vi "GVSGet QueueName From DataView Idx.vi"(11 "DataView Idx":i32) -> (3 "DataView sQueueName":string)   [LabVIEW 2013]
uses:
  GVSNew View Global.vi
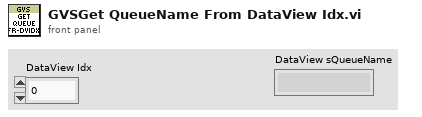
[diagram p1: front panel]
types:
  T1 = typedef "Graph Main Info Cluster.ctl" = cluster{"Selected_BarIdx":i32, "Selected_PanelIdx":i32, "Graph Main VIRef":refnum<vi>, "ToolBarClick":bool, "Spliter Ref Array":refnum<vi>[], "Panel Ref Array":refnum<vi>[], "Spliter_matrix":i32[][], "Panel_matrix":i32[][], "child_spliterIdx_matrix":i32[][], "split_pos_matrix":i32[][], "Title State":bool, "sQueueName":string, "Frame nID":i32, "Graph VIRef Array":cluster{"Graph VIRef":refnum<vi>, "Panel Idx":i32, "Frame VIRef":refnum<vi>, "Icon Ring":i32, "Graph Type":string}[], "View Type":string}
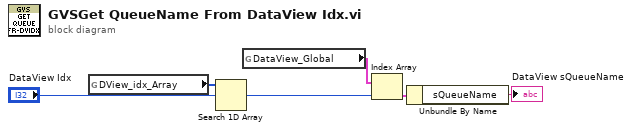
[diagram p0: block diagram]
diagram:
  n1 = global read "GVSNew View Global.vi" "DView_idx_Array"() -> (w6:i32[])
  n2 = Search 1D Array(1D array=w6, element="DataView Idx") -> (index of element=w3:i32)  [unwired: 1 in]
  n3 = global read "GVSNew View Global.vi" "DataView_Global"() -> (w4:T1[])
  n4 = Index Array(array=w4, index=w3) -> (element=w2:T1)
  n5 = Unbundle By Name(w2) -> ("sQueueName"=→"DataView sQueueName":string)
